vi "ParseString.vi"(11 "String":string) -> (3 "Array":string[](array[string]))   [LabVIEW 2016]
doc: "Turns a string of tokens seperated by commas into an array of the tokens"
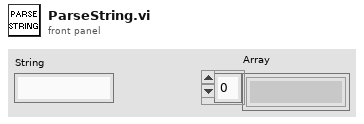
[diagram p1: front panel]
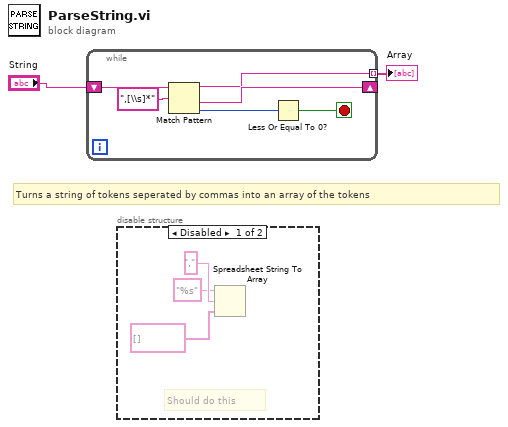
[diagram p0: block diagram]
diagram:
  # "Turns a string of tokens seperated by commas into an array of the tokens"
  n1 = while {
    shift-right: [w7] -> _
    shift-left: "String" -> [w8]
    tunnel: [w4] -> w1 mode=indexing
    stop <- w5 stop-if-true
    n2 = Match Pattern(string=w8, regular expression=",[\\s]*") -> (before substring=w4:string, after substring=w7:string, offset past match=w6:i32)  [unwired: 1 in, 1 out]
    n3 = Less Or Equal To 0?(x=w6) -> (x <= 0?=w5:bool)
  }
  "Array" <- w1
  n4 = disable-structure shown="Disabled" {
    frame Disabled {
      # "Should do this"
      n5 = Spreadsheet String To Array(delimiter (Tab)=",", format string="%s", array type (2D Dbl)=string[] [] ("Array 2")) -> ()  [unwired: 1 in, 1 out]
    }
    frame Enabled {
    }
  }
